vi "DSF.Engine.BuilderManager.Get Builder States Pointer.vi"(11 "Builder Manager in":refnum<class "DSF.Engine.BuilderManager.lvclass">) -> (2 "Builder States":refnum<class "DSF.Engine.Pointer.Status.Builder.State.lvclass">, 3 "Builder Manager out":refnum<class "DSF.Engine.BuilderManager.lvclass">)   [LabVIEW 2016, in "DSF.Engine.lvlib" / "DSF.Engine.BuilderManager.lvclass"]
uses:
  DSF.Engine.BuilderManager.lvclass
  Pointer/DSF.Engine.Pointer.Status.Builder.State.lvclass
  DSF.Engine.BuilderManager.lvclass/DSF.Engine.BuilderManager.ctl
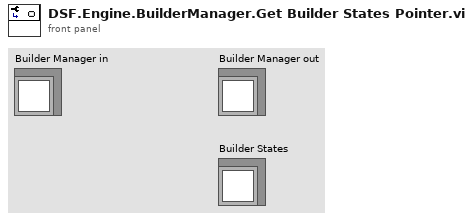
[diagram p1: front panel]
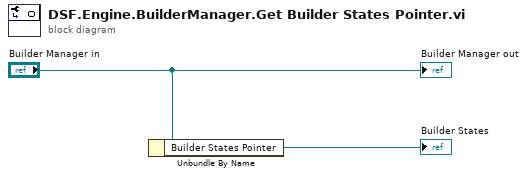
[diagram p0: block diagram]
diagram:
  n1 = Unbundle By Name("Builder Manager in") -> ("Builder States Pointer"=→"Builder States":refnum<class "DSF.Engine.Pointer.Status.Builder.State.lvclass">)
  "Builder Manager out" <- "Builder Manager in"
